vi "Read Multi Eval Meas Trace IEM Results.vi"(8 "error in (no error)":errorcluster, 9 "ResultType (Current)":i32(ring) items=["Current", "Average", "Maximum"], 10 "Instance (1)":T1=1, 11 "VISA resource name":refnum<visa-resource-name>) -> (0 "error out":errorcluster, 1 "Trace IEM Results":dbl[](array[numeric]) format="%^.3e", 2 "Reliability":i32, 3 "VISA resource name out":refnum<visa-resource-name>)   [LabVIEW 2020, in "Rohde&Schwarz CMXP NR FR2 Measurement.lvlib"]
doc: "Starts a new single shot measurement and returns the multi eval measurement IEM trace results.\n\nAttributes:\nRSCMXPNRFR2M_ATTR_READ_MULTI_EVAL_MEASUREMENT_TRACE_IEM_AVERAGE_RESULTS\nRSCMXPNRFR2M_ATTR_READ_MULTI_EVAL_MEASUREMENT_TRACE_IEM_CURRENT_RESULTS\nRSCMXPNRFR2M_ATTR_READ_MULTI_EVAL_MEASUREMENT_TRACE_IEM_MAXIMUM_RESULTS\n\nRemote-control commands:\nREAD:NRMMw:MEAS<i>:MEValuation:TRACe:IEMissions:AVERage?\nREAD:NRMMw:MEAS<i>:MEValuation:TRACe:IEMissions:CURRent?\nREAD:NRMMw:MEAS<i>:MEValuation:TRACe:IEMissions:MAXimum?"
uses:
  <instrlib>/Rohde&Schwarz CMXP NR FR2 Measurement/Rohde&Schwarz CMXP NR FR2 Measurement.lvlib
  <instrlib>/Rohde&Schwarz CMXP NR FR2 Measurement/Private/_Instance.ctl
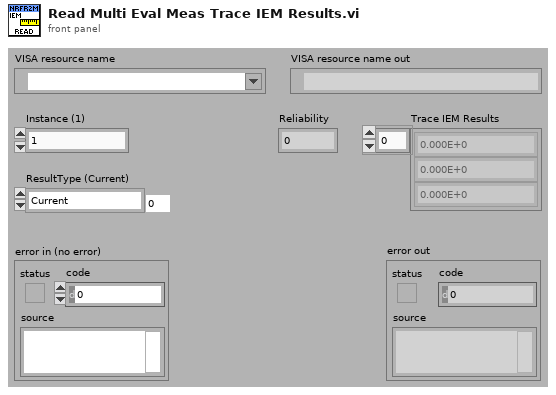
[diagram p1: front panel]
types:
  T1 = typedef "Rohde&Schwarz CMXP NR FR2 Measurement.lvlib/_Instance.ctl" = i32
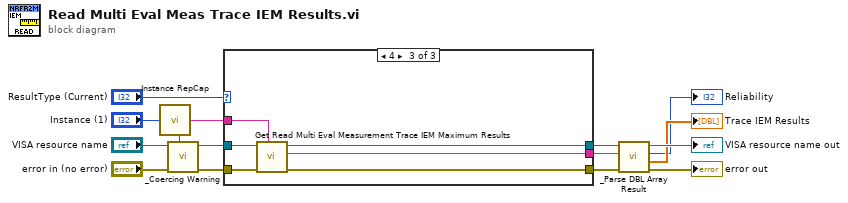
[diagram p0: block diagram]
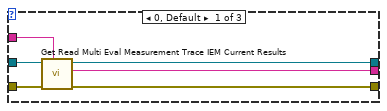
[diagram p2: hidden frame]
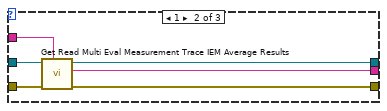
[diagram p3: hidden frame]
diagram:
  n1 = call <instrlib>:"Instance RepCap.vi"("Instance In"="Instance (1)") -> ("In Range?"=w7:bool, "RepCap Identifier Out"=w15:string)  [unwired: 1 in]
  n2 = call <instrlib>:"_Coercing Warning.vi"("In Range?"=w7, "error in (no error)"="error in (no error)", "VISA resource name"="VISA resource name") -> ("error out"=w5:errorcluster, "VISA resource name out"=w6:refnum<visa-resource-name>)  [unwired: 7 in]
  n3 = case shown="4" "ResultType (Current)" {
    tunnel: w15 -> [w21 w27 w33]
    tunnel: [w20 w26 w32] -> w14
    tunnel: [w19 w25 w31] -> w13
    tunnel: [w18 w24 w30] -> w10
    tunnel: w5 -> [w17 w23 w29]
    tunnel: w6 -> [w16 w22 w28]
    frame 0, Default {
      n4 = call "Get Read Multi Eval Measurement Trace IEM Current Results"("Repeated Capabilities"=w21, "error in (no error)"=w17, "instrument handle"=w16) -> ("error out"=w20:errorcluster, "Read Multi Eval Measurement Trace IEM Current Results"=w18:string, "instrument handle out"=w19:refnum<visa-resource-name>)  [unwired: 6 in]
    }
    frame 1 {
      n5 = call "Get Read Multi Eval Measurement Trace IEM Average Results"("Repeated Capabilities"=w27, "error in (no error)"=w23, "instrument handle"=w22) -> ("error out"=w26:errorcluster, "Read Multi Eval Measurement Trace IEM Average Results"=w24:string, "instrument handle out"=w25:refnum<visa-resource-name>)  [unwired: 6 in]
    }
    frame 4 {
      n6 = call "Get Read Multi Eval Measurement Trace IEM Maximum Results"("Repeated Capabilities"=w33, "error in (no error)"=w29, "instrument handle"=w28) -> ("error out"=w32:errorcluster, "Read Multi Eval Measurement Trace IEM Maximum Results"=w30:string, "instrument handle out"=w31:refnum<visa-resource-name>)  [unwired: 6 in]
    }
  }
  n7 = call <instrlib>:"_Parse DBL Array Result.vi"("error in (no error)"=w14, "Input String"=w10, "VISA resource name"=w13) -> ("error out"=→"error out":errorcluster, "Results"=→"Trace IEM Results":dbl[], "Reliability"=→"Reliability":i32, "VISA resource name out"=→"VISA resource name out":refnum<visa-resource-name>)  [unwired: 5 in]
